vi "Actor Core.vi"(8 "error in":errorcluster, 11 "Virtual Camera in":refnum<class "Virtual Camera.lvclass">) -> (0 "error out":errorcluster, 3 "Actor out":refnum<class "Actor.lvclass">)   [LabVIEW 2018, in "Virtual Camera.lvlib" / "Virtual Camera.lvclass"]
doc: "(<B>Filename</B>: Actor Framework.lvlib:Actor.lvclass:Actor Core.vi)\n\nReceives messages to the actor, reacts to them, and initiates any error handling that may shut the actor down.\n\nDescendant classes may override this VI to append parallel tasks for the actor to complete while it handles messages. Overrides use the Call Parent Method node."
uses:
  Virtual Camera.lvclass
  C:/Program Files/National Instruments/LabVIEW 2018/vi.lib/ActorFramework/Actor/Actor.lvclass
  <vilib>/ActorFramework/Actor/Actor.lvclass
  <vilib>/ActorFramework/Actor/Actor.lvclass/Actor.ctl
  <vilib>/ActorFramework/Message Enqueuer/Message Enqueuer.lvclass/Message Enqueuer.ctl
  <vilib>/ActorFramework/Message Enqueuer/Enqueue.vi
  Application Messages/Record Button Off Msg/Record Button Off Msg.lvclass
  C:/Program Files/National Instruments/LabVIEW 2018/vi.lib/ActorFramework/Message/Message.lvclass
  Resources/GLOBAL/GLOBAL Time-critical.vi
  <vilib>/ActorFramework/Message Priority Queue/Priority Enqueue.vi
  Camera/Camera.lvclass
panel:
  in  "Stop Button":bool
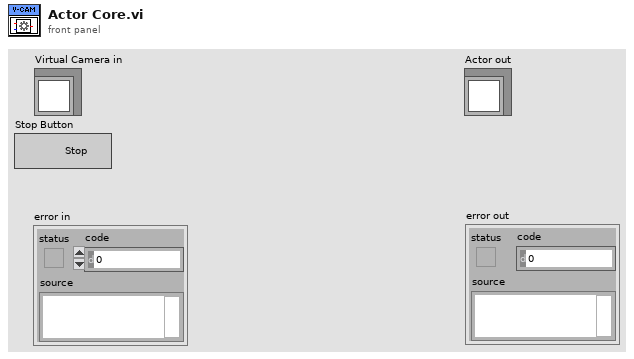
[diagram p1: front panel]
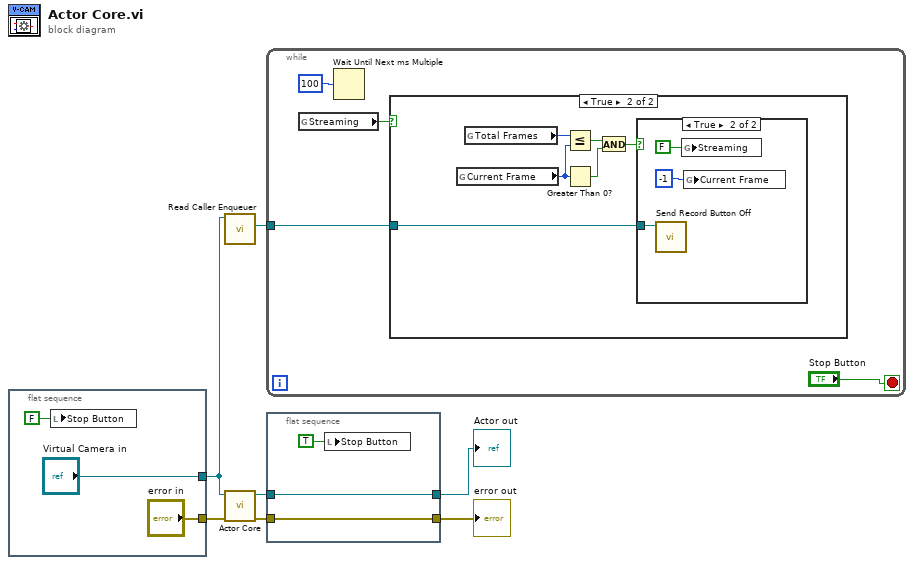
[diagram p0: block diagram]
diagram:
  n1 = flat-sequence {
    tunnel: ["error in"] -> w7
    tunnel: ["Virtual Camera in"] -> w2
    frame #0 {
      n2 = local write "Stop Button"(FALSE ("Stop Button")) -> ()
    }
  }
  n3 = call <vilib>:"Read Caller Enqueuer.vi"("Actor"=w2) -> ("Caller Enqueuer"=w1:refnum<class "Message Enqueuer.lvclass">)  [unwired: 10 in]
  n4 = call-parent "Actor Core.vi"("error in"=w7, "Device in"=w2) -> ("error out"=w4:errorcluster, "Actor out"=w6:refnum<class "Actor.lvclass">)  [unwired: 8 in]
  n5 = while {
    tunnel: w1 -> [w11]
    stop <- "Stop Button" stop-if-true
    n6 = global read "GLOBAL Time-critical.vi" "Streaming"() -> (w12:bool)
    n7 = Wait Until Next ms Multiple(millisecond multiple=u32 100) -> ()  [unwired: 1 out]
    n8 = case shown="True" w12 {
      tunnel: w11 -> [_ w15]
      frame False {
      }
      frame True {
        n9 = global read "GLOBAL Time-critical.vi" "Current Frame"() -> (w16:i32)
        n10 = global read "GLOBAL Time-critical.vi" "Total Frames"() -> (w20:i32)
        n11 = Less Or Equal?(x=w20, y=w16) -> (x <= y?=w19:bool)
        n12 = Greater Than 0?(x=w16) -> (x > 0?=w18:bool)
        n13 = And(x=w19, y=w18) -> (x .and. y?=w17:bool)
        n14 = case shown="True" w17 {
          tunnel: w15 -> [_ w23]
          frame False {
          }
          frame True {
            n15 = call "Send Record Button Off.vi"("Message Enqueuer"=w23) -> ()  [unwired: 9 in, 2 out]
            n16 = global write "GLOBAL Time-critical.vi" "Streaming"(FALSE ("Streaming")) -> ()
            n17 = global write "GLOBAL Time-critical.vi" "Current Frame"(-1 ("Current Frame")) -> ()
          }
        }
      }
    }
  }
  n18 = flat-sequence {
    tunnel: w6 -> [w25]
    tunnel: [w25] -> w5
    tunnel: w4 -> [w24]
    tunnel: [w24] -> w3
    frame #0 {
      n19 = local write "Stop Button"(TRUE ("Stop Button")) -> ()
    }
  }
  "error out" <- w3
  "Actor out" <- w5
